vi "Close TDMS.vi"(8 "error in (no error)":errorcluster, 11 "Maxon Encoder in":refnum<class "Maxon Encoder.lvclass">) -> (0 "error out":errorcluster, 3 "Maxon Encoder out":refnum<class "Maxon Encoder.lvclass">)   [LabVIEW 2019, in "Maxon Encoder.lvclass"]
doc: "Closes the tdms file."
uses:
  Maxon Encoder.lvclass
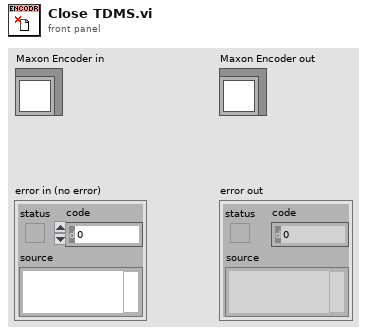
[diagram p1: front panel]
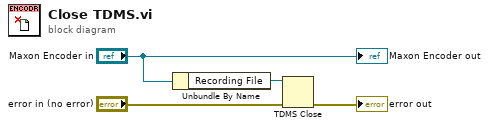
[diagram p0: block diagram]
diagram:
  n1 = Unbundle By Name("Maxon Encoder in") -> ("Recording File"=w4:refnum<k34>)
  n2 = TDMS Close(8:"error in (no error)", 11:w4) -> (0:→"error out":errorcluster)  [unwired: 1 out]
  "Maxon Encoder out" <- "Maxon Encoder in"
